vi "SwerveDriveFace.vi"(8 "error in (no error)":errorcluster, 9 "Face Joystick Axes":cluster{"X":dbl, "Y":dbl}, 10 "Strafe Joystick Axes":cluster{"X":dbl, "Y":dbl}, 11 "Gyro refnum name":string="My Gyro RefNum") -> (0 "error out":errorcluster)   [LabVIEW 2014]
uses:
  <vilib>/addons/control/pid/pid.llb/PID Control Input Filter (DBL).vi
  <vilib>/addons/control/pid/pid.llb/PID (DBL).vi
  Robot Global Data.vi
  <vilib>/addons/control/pid/NI_PID_pid.lvlib
panel:
  in  "Face PID Gains":T1={"proportional gain (Kc)"=1.0, "integral time (Ti, min)"=0.01, "derivative time (Td, min)"=0.0} {"derivative time (Td, min)" format="%.3f"; "integral time (Ti, min)" format="%.3f"; "proportional gain (Kc)" format="%.3f"}
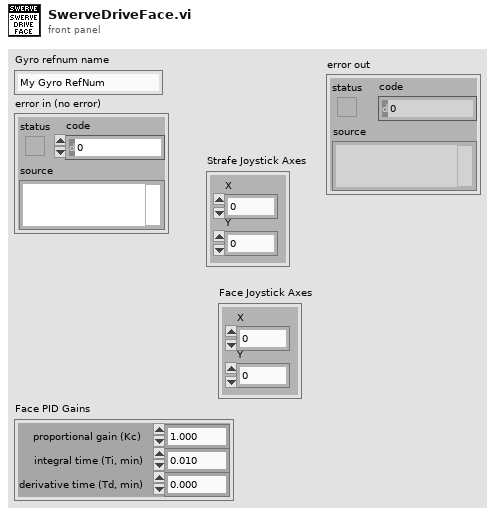
[diagram p1: front panel]
types:
  T1 = cluster{"proportional gain (Kc)":dbl, "integral time (Ti, min)":dbl, "derivative time (Td, min)":dbl}
  T2 = typedef "WPI_GyroDevRef.ctl" = cluster{"DevStatus":errorcluster, "Analog Module":T3, "Analog Channel":T4, "Offset":dbl, "Gain (VoltsPerDegree/Second)":dbl}
  T3 = typedef "FPGA_TypedefAnalogModule.ctl" = enum16{"Controller 1"}
  T4 = typedef "FPGA_AIChannel.ctl" = enum8{"AI 0", "AI 1", "AI 2", "AI 3", "AI MXP 0", "AI MXP 1", "AI MXP 2", "AI MXP 3", "Invalid"}
  T5 = typedef "WPI_MotorControlDeviceRef.ctl" = cluster{"DeviceStatus":errorcluster, "Type":T6, "PWM":cluster{"Controller":T7, "PWM Channel":T8, "DeadBand":T9}, "CAN":cluster{"Device Number":u8, "Control Mode":T10, "Semaphore":T11, "Max Vout":dbl, "TalonSRX Control Mode":T12}, "Invert":bool, "TransformRef":T13, "InvTransformRef":T13}
  T6 = typedef "WPI_MotorControlType.ctl" = enum16{"PWM", "CAN", "CANTalonSRX"}
  T7 = typedef "FPGA_TypedefDigitalModule.ctl" = enum16{"Controller 1"}
  T8 = typedef "FPGA_DIOPWMChannel.ctl" = enum8{"PWM 0", "PWM 1", "PWM 2", "PWM 3", "PWM 4", "PWM 5", "PWM 6", "PWM 7", "PWM 8", "PWM 9", "PWM MXP 0", "PWM MXP 1", "PWM MXP 2", "PWM MXP 3", "PWM MXP 4", "PWM MXP 5", "PWM MXP 6", "PWM MXP 7", "PWM MXP 8", "PWM MXP 9", "Invalid"}
  T9 = typedef "WPI_PWMDeadband.ctl" = cluster{"Name":string, "maxPositivePwm":i32, "minPositivePwm":i32, "centerPwm":i32, "maxNegativePwm":i32, "minNegativePwm":i32, "angularRange":u16}
  T10 = typedef "WPI_CANJaguar_ControlMode.ctl" = enum8{"Percent VBus", "Current", "Speed", "Position", "Voltage"}
  T11 = typedef "Semaphore RefNum" = refnum<k1>
  T12 = typedef "WPI_CANTalonSRX_APIControlMode.ctl" = enum8{"Percent VBus", "Speed", "Position", "Slave", "Unchanged / Invalid"}
  T13 = typedef "WPI_PWMTransform_ConPane.ctl" = refnum<vi>
  T14 = typedef "WPI_CANTalonSRX_GlobalStatus.ctl" = cluster{"Applied Throttle":dbl, "Module Enabled":bool, "CAN Error":errorcluster, "Closed Loop Error":dbl, "Forward Limit Switch Closed":bool, "Reverse Limit Switch Closed":bool, "Sensor Position":dbl, "Sensor Velocity":dbl, "Current":dbl, "Sticky Fault - Over Temp":bool, "Sticky Fault - Under Voltage":bool, "Sticky Fault - Forward Limit":bool, "Sticky Fault - Reverse Limit":bool, "Sticky Fault - Forward Soft Limit":bool, "Sticky Fault - Reverse Soft Limit":bool, "Brake is Enabled":bool, "Encoder Position":dbl, "Encoder Velocity":dbl, "Encoder Index Count":dbl, "Encoder A Pin State":bool, "Encoder B Pin State":bool, "Encoder Index Pin State":bool, "Analog In":dbl, "Analog In Velocity":dbl, "Temperature (C)":dbl, "Battery Voltage":dbl}
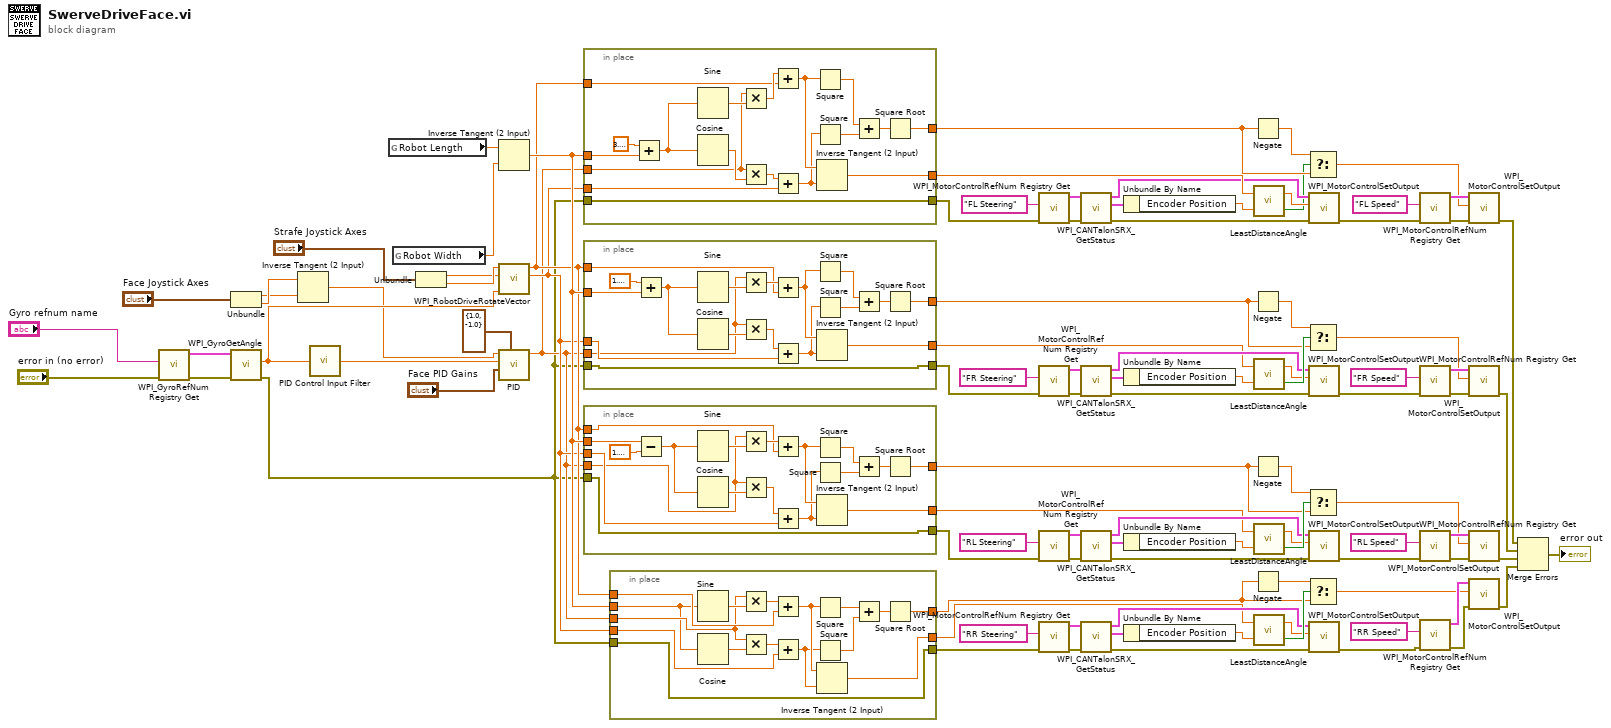
[diagram p0: block diagram]
diagram:
  n1 = call <vilib>:"WPI_GyroRefNum Registry Get.vi"("error in (no error)"="error in (no error)", "refnum name"="Gyro refnum name") -> ("error out"=w57:errorcluster, "GyroDevRef"=w56:T2)  [unwired: 8 in]
  n2 = Unbundle("Face Joystick Axes") -> ("X"=w49:dbl, "Y"=w50:dbl)
  n3 = call <vilib>:"WPI_GyroGetAngle.vi"("error in (no error)"=w57, "GyroDevRef"=w56) -> ("error out"=w63:errorcluster, "Angle"=w99:dbl)  [unwired: 6 in, 2 out]
  n4 = Inverse Tangent (2 Input)(1:w49, 2:w50) -> (0:w52:dbl)
  n5 = call-poly <vilib>:"PID Control Input Filter.vi"("input"=w99) -> ("output"=w55:dbl)  [unwired: 4 in]
  n6 = global read "Robot Global Data.vi" "Robot Length"() -> (w97:dbl)
  n7 = global read "Robot Global Data.vi" "Robot Width"() -> (w98:dbl)
  n8 = Unbundle("Strafe Joystick Axes") -> ("X"=w83:dbl, "Y"=w84:dbl)
  n9 = Inverse Tangent (2 Input)(1:w98, 2:w97) -> (0:w68:dbl)
  n10 = call <vilib>:"WPI_RobotDriveRotateVector.vi"("Angle"=w99, "X"=w83, "Y"=w84) -> ("X'"=w66:dbl, "Y'"=w67:dbl)  [unwired: 7 out]
  n11 = call-poly <vilib>:"PID.vi"("output range"=cluster{"output high":dbl, "output low":dbl} {"output high"=1.0, "output low"=-1.0}, "PID gains"="Face PID Gains", "process variable"=w55, "setpoint"=w52) -> ("output"=w65:dbl)  [unwired: 6 in, 1 out]
  n12 = in-place {
    in-place-border: w67 -> [w106]
    in-place-border: w66 -> [w108]
    in-place-border: w65 -> [w101]
    in-place-border: w68 -> [w111]
    in-place-border: [w103] -> w46
    in-place-border: [w102] -> w39
    in-place-border: w63 -> [w100]
    in-place-border: [w100] -> w62
    n13 = Add(x=3.141592653589793, y=w111) -> (x+y=w110:dbl)
    n14 = Sine(x=w110) -> (sin(x)=w114:dbl)
    n15 = Cosine(x=w110) -> (cos(x)=w113:dbl)
    n16 = Multiply(x=w101, y=w114) -> (x*y=w107:dbl)
    n17 = Multiply(x=w101, y=w113) -> (x*y=w109:dbl)
    n18 = Add(x=w107, y=w106) -> (x+y=w105:dbl)
    n19 = Add(x=w109, y=w108) -> (x+y=w104:dbl)
    n20 = Square(x=w105) -> (x^2=w116:dbl)
    n21 = Square(x=w104) -> (x^2=w115:dbl)
    n22 = Inverse Tangent (2 Input)(1:w104, 2:w105) -> (0:w103:dbl)
    n23 = Add(x=w116, y=w115) -> (x+y=w117:dbl)
    n24 = Square Root(x=w117) -> (sqrt(x)=w102:dbl)
  }
  n25 = in-place {
    in-place-border: w67 -> [w124]
    in-place-border: w66 -> [w126]
    in-place-border: w65 -> [w119]
    in-place-border: w68 -> [w129]
    in-place-border: [w121] -> w26
    in-place-border: [w120] -> w28
    in-place-border: w63 -> [w118]
    in-place-border: [w118] -> w61
    n26 = Add(x=1.5707963267948966, y=w129) -> (x+y=w128:dbl)
    n27 = Sine(x=w128) -> (sin(x)=w132:dbl)
    n28 = Cosine(x=w128) -> (cos(x)=w131:dbl)
    n29 = Multiply(x=w119, y=w132) -> (x*y=w125:dbl)
    n30 = Multiply(x=w119, y=w131) -> (x*y=w127:dbl)
    n31 = Add(x=w125, y=w124) -> (x+y=w123:dbl)
    n32 = Add(x=w127, y=w126) -> (x+y=w122:dbl)
    n33 = Square(x=w123) -> (x^2=w134:dbl)
    n34 = Square(x=w122) -> (x^2=w133:dbl)
    n35 = Inverse Tangent (2 Input)(1:w122, 2:w123) -> (0:w121:dbl)
    n36 = Add(x=w134, y=w133) -> (x+y=w135:dbl)
    n37 = Square Root(x=w135) -> (sqrt(x)=w120:dbl)
  }
  n38 = in-place {
    in-place-border: w67 -> [w145]
    in-place-border: w66 -> [w147]
    in-place-border: w65 -> [w140]
    in-place-border: w68 -> [w139]
    in-place-border: [w142] -> w16
    in-place-border: [w141] -> w14
    in-place-border: w63 -> [w136]
    in-place-border: [w136] -> w60
    n39 = Subtract(x=w139, y=1.5707963267948966) -> (x-y=w137:dbl)
    n40 = Sine(x=w137) -> (sin(x)=w150:dbl)
    n41 = Cosine(x=w137) -> (cos(x)=w149:dbl)
    n42 = Multiply(x=w140, y=w150) -> (x*y=w146:dbl)
    n43 = Multiply(x=w140, y=w149) -> (x*y=w148:dbl)
    n44 = Add(x=w146, y=w145) -> (x+y=w144:dbl)
    n45 = Add(x=w148, y=w147) -> (x+y=w143:dbl)
    n46 = Square(x=w144) -> (x^2=w152:dbl)
    n47 = Square(x=w143) -> (x^2=w151:dbl)
    n48 = Inverse Tangent (2 Input)(1:w143, 2:w144) -> (0:w142:dbl)
    n49 = Add(x=w152, y=w151) -> (x+y=w153:dbl)
    n50 = Square Root(x=w153) -> (sqrt(x)=w141:dbl)
  }
  n51 = in-place {
    in-place-border: w67 -> [w161]
    in-place-border: w66 -> [w163]
    in-place-border: w65 -> [w156]
    in-place-border: w68 -> [w155]
    in-place-border: [w158] -> w4
    in-place-border: [w157] -> w2
    in-place-border: w63 -> [w154]
    in-place-border: [w154] -> w59
    n52 = Sine(x=w155) -> (sin(x)=w166:dbl)
    n53 = Cosine(x=w155) -> (cos(x)=w165:dbl)
    n54 = Multiply(x=w156, y=w166) -> (x*y=w162:dbl)
    n55 = Multiply(x=w156, y=w165) -> (x*y=w164:dbl)
    n56 = Add(x=w162, y=w161) -> (x+y=w160:dbl)
    n57 = Add(x=w164, y=w163) -> (x+y=w159:dbl)
    n58 = Square(x=w160) -> (x^2=w168:dbl)
    n59 = Square(x=w159) -> (x^2=w167:dbl)
    n60 = Inverse Tangent (2 Input)(1:w159, 2:w160) -> (0:w158:dbl)
    n61 = Add(x=w168, y=w167) -> (x+y=w169:dbl)
    n62 = Square Root(x=w169) -> (sqrt(x)=w157:dbl)
  }
  n63 = call <vilib>:"WPI_MotorControlRefNum Registry Get.vi"("error in (no error)"=w62, "refnum name"="FL Steering") -> ("error out"=w44:errorcluster, "MotorControlDevRef"=w94:T5)  [unwired: 8 in]
  n64 = call <vilib>:"WPI_MotorControlRefNum Registry Get.vi"("error in (no error)"=w61, "refnum name"="FR Steering") -> ("error out"=w31:errorcluster, "MotorControlDevRef"=w32:T5)  [unwired: 8 in]
  n65 = call <vilib>:"WPI_MotorControlRefNum Registry Get.vi"("error in (no error)"=w60, "refnum name"="RL Steering") -> ("error out"=w17:errorcluster, "MotorControlDevRef"=w18:T5)  [unwired: 8 in]
  n66 = call <vilib>:"WPI_MotorControlRefNum Registry Get.vi"("error in (no error)"=w59, "refnum name"="RR Steering") -> ("error out"=w7:errorcluster, "MotorControlDevRef"=w8:T5)  [unwired: 8 in]
  n67 = call <vilib>:"WPI_CANTalonSRX_GetStatus.vi"("error in (no error)"=w44, "CAN Talon SRX Ref"=w94) -> ("error out"=w43:errorcluster, "Talon SRX Status"=w42:T14, "CAN Talon SRX Ref Out"=w45:T5)  [unwired: 7 in]
  n68 = call <vilib>:"WPI_CANTalonSRX_GetStatus.vi"("error in (no error)"=w31, "CAN Talon SRX Ref"=w32) -> ("error out"=w29:errorcluster, "Talon SRX Status"=w36:T14, "CAN Talon SRX Ref Out"=w30:T5)  [unwired: 7 in]
  n69 = call <vilib>:"WPI_CANTalonSRX_GetStatus.vi"("error in (no error)"=w17, "CAN Talon SRX Ref"=w18) -> ("error out"=w20:errorcluster, "Talon SRX Status"=w24:T14, "CAN Talon SRX Ref Out"=w19:T5)  [unwired: 7 in]
  n70 = call <vilib>:"WPI_CANTalonSRX_GetStatus.vi"("error in (no error)"=w7, "CAN Talon SRX Ref"=w8) -> ("error out"=w6:errorcluster, "Talon SRX Status"=w12:T14, "CAN Talon SRX Ref Out"=w5:T5)  [unwired: 7 in]
  n71 = Unbundle By Name(w42) -> ("Encoder Position"=w41:dbl)
  n72 = Unbundle By Name(w36) -> ("Encoder Position"=w35:dbl)
  n73 = Unbundle By Name(w24) -> ("Encoder Position"=w23:dbl)
  n74 = Unbundle By Name(w12) -> ("Encoder Position"=w11:dbl)
  n75 = Negate(x=w39) -> (-x=w38:dbl)
  n76 = Negate(x=w28) -> (-x=w34:dbl)
  n77 = Negate(x=w14) -> (-x=w22:dbl)
  n78 = Negate(x=w2) -> (-x=w10:dbl)
  n79 = call "LeastDistanceAngle.vi"("current angle (no limits)"=w41, "target angle (between pi and -pi)"=w46) -> ("Reverse?"=w37:bool, "motor output angle"=w47:dbl)
  n80 = call "LeastDistanceAngle.vi"("current angle (no limits)"=w35, "target angle (between pi and -pi)"=w26) -> ("Reverse?"=w33:bool, "motor output angle"=w25:dbl)
  n81 = call "LeastDistanceAngle.vi"("current angle (no limits)"=w23, "target angle (between pi and -pi)"=w16) -> ("Reverse?"=w21:bool, "motor output angle"=w15:dbl)
  n82 = call "LeastDistanceAngle.vi"("current angle (no limits)"=w11, "target angle (between pi and -pi)"=w4) -> ("Reverse?"=w9:bool, "motor output angle"=w3:dbl)
  n83 = Select(t=w38, s=w37, f=w39) -> (s? t:f=w40:dbl)
  n84 = Select(t=w34, s=w33, f=w28) -> (s? t:f=w27:dbl)
  n85 = Select(t=w22, s=w21, f=w14) -> (s? t:f=w13:dbl)
  n86 = Select(t=w10, s=w9, f=w2) -> (s? t:f=w1:dbl)
  n87 = call <vilib>:"WPI_MotorControlSetOutput.vi"("error in (no error)"=w43, "Output"=w47, "MotorControlDevRef"=w45) -> ("error out"=w91:errorcluster)  [unwired: 6 in, 2 out]
  n88 = call <vilib>:"WPI_MotorControlSetOutput.vi"("error in (no error)"=w29, "Output"=w25, "MotorControlDevRef"=w30) -> ("error out"=w86:errorcluster)  [unwired: 6 in, 2 out]
  n89 = call <vilib>:"WPI_MotorControlSetOutput.vi"("error in (no error)"=w20, "Output"=w15, "MotorControlDevRef"=w19) -> ("error out"=w75:errorcluster)  [unwired: 6 in, 2 out]
  n90 = call <vilib>:"WPI_MotorControlSetOutput.vi"("error in (no error)"=w6, "Output"=w3, "MotorControlDevRef"=w5) -> ("error out"=w69:errorcluster)  [unwired: 6 in, 2 out]
  n91 = call <vilib>:"WPI_MotorControlRefNum Registry Get.vi"("error in (no error)"=w91, "refnum name"="FL Speed") -> ("error out"=w93:errorcluster, "MotorControlDevRef"=w92:T5)  [unwired: 8 in]
  n92 = call <vilib>:"WPI_MotorControlRefNum Registry Get.vi"("error in (no error)"=w86, "refnum name"="FR Speed") -> ("error out"=w88:errorcluster, "MotorControlDevRef"=w87:T5)  [unwired: 8 in]
  n93 = call <vilib>:"WPI_MotorControlRefNum Registry Get.vi"("error in (no error)"=w75, "refnum name"="RL Speed") -> ("error out"=w77:errorcluster, "MotorControlDevRef"=w76:T5)  [unwired: 8 in]
  n94 = call <vilib>:"WPI_MotorControlRefNum Registry Get.vi"("error in (no error)"=w69, "refnum name"="RR Speed") -> ("error out"=w71:errorcluster, "MotorControlDevRef"=w70:T5)  [unwired: 8 in]
  n95 = call <vilib>:"WPI_MotorControlSetOutput.vi"("error in (no error)"=w93, "Output"=w40, "MotorControlDevRef"=w92) -> ("error out"=w80:errorcluster)  [unwired: 6 in, 2 out]
  n96 = call <vilib>:"WPI_MotorControlSetOutput.vi"("error in (no error)"=w88, "Output"=w27, "MotorControlDevRef"=w87) -> ("error out"=w82:errorcluster)  [unwired: 6 in, 2 out]
  n97 = call <vilib>:"WPI_MotorControlSetOutput.vi"("error in (no error)"=w77, "Output"=w13, "MotorControlDevRef"=w76) -> ("error out"=w74:errorcluster)  [unwired: 6 in, 2 out]
  n98 = call <vilib>:"WPI_MotorControlSetOutput.vi"("error in (no error)"=w71, "Output"=w1, "MotorControlDevRef"=w70) -> ("error out"=w64:errorcluster)  [unwired: 6 in, 2 out]
  n99 = Merge Errors(w80, w82, w74, w64) -> (→"error out":errorcluster)
